vi "Purge.vi"(5 "Digital I/O Pin":u8=7, 7 "Arduino Resource":T1={"VISA resource"="GlueCTRL", "Board Type"=enum."Uno", "Connection Type"=enum."USB / Serial", "Bytes Per Packet (15)"=15}, 8 "Pin Down?":bool=TRUE, 9 "Axis Speeds":T3={"X [mm/s]"=25.0, "Y [mm/s]"=25.0, "Z [mm/s]"=10.0}, 10 "Start Position [mm]":dbl[](array[numeric]), 11 ".NET Refnum In":refnum<k24>) -> ()   [LabVIEW 2016]
uses:
  C:/Users/Aerotech/Documents/BNLStaveAssembly-blueprint/Bin/Aerotech.A3200.dll
  BNLStaveAssembly-blueprint/Bin/Aerotech.A3200.dll
  <vilib>/LabVIEW Interface for Arduino/Type Defs/Arduino Resource.ctl
  <vilib>/LabVIEW Interface for Arduino/Type Defs/Board Type.ctl
  <vilib>/LabVIEW Interface for Arduino/LabVIEW Interface for Arduino.lvlib
panel:
  in  "Absolute Purge Height [mm]":dbl=-30.0 format="%#_13g"
  in  "Relative Change in X, Y to Purge [mm]":dbl[](array[numeric])=[0.0, -150.0, 0.0]
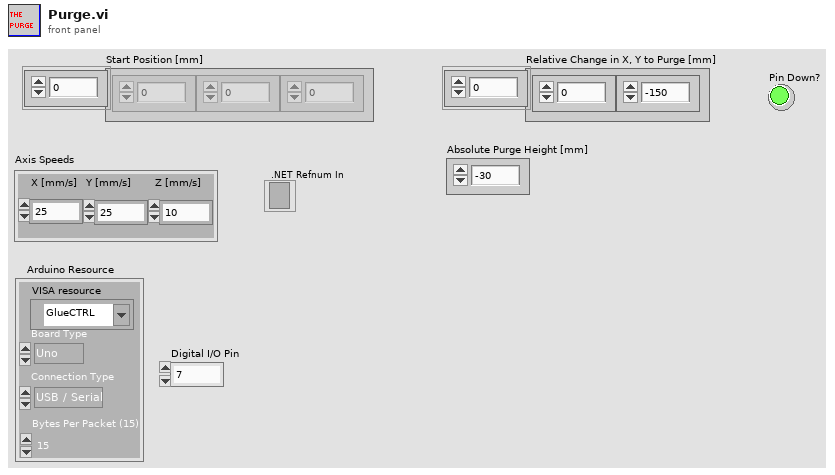
[diagram p1: front panel]
types:
  T1 = typedef "LabVIEW Interface for Arduino.lvlib/Arduino Resource.ctl" = cluster{"VISA resource":refnum<visa-resource-name>, "Board Type":T2, "Connection Type":enum8{"USB / Serial"}, "Bytes Per Packet (15)":u8}
  T2 = typedef "LabVIEW Interface for Arduino.lvlib/Board Type.ctl" = enum16{"Uno", "Dimuelanove w/Atmega 328", "Mega 2560"}
  T3 = cluster{"X [mm/s]":dbl, "Y [mm/s]":dbl, "Z [mm/s]":dbl}
  T4 = cluster{"Start Position [mm][0]":dbl, "Start Position [mm][1]":dbl, "Start Position [mm][2]":dbl}
  T5 = cluster{"Final X":dbl, "Final Y":dbl, "Final Z":dbl}
  T6 = cluster{"Final Position[0]":dbl, "Final Position[1]":dbl, "Final Position[2]":dbl}
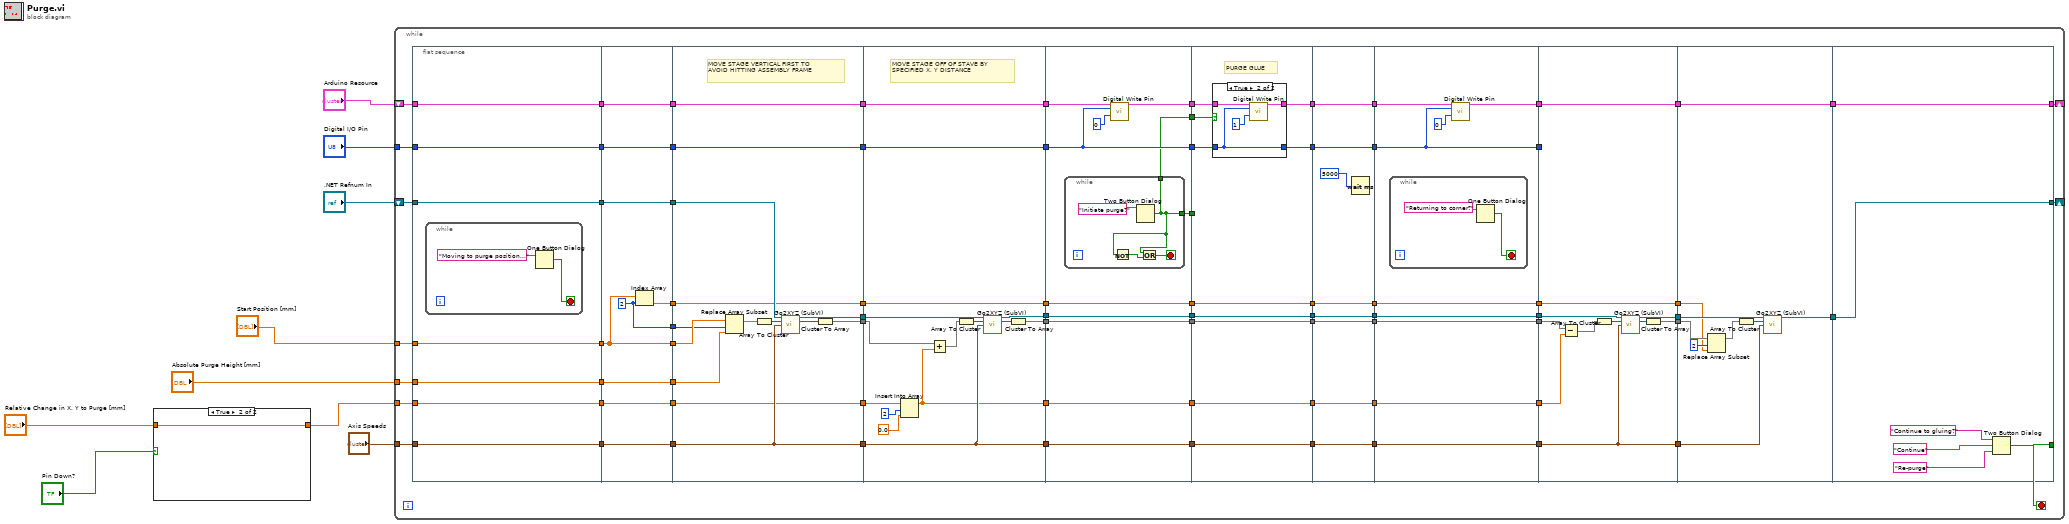
[diagram p0: block diagram]
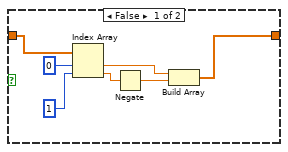
[diagram p2: hidden frame]
diagram:
  n1 = case shown="True" "Pin Down?" {
    tunnel: "Relative Change in X, Y to Purge [mm]" -> [w16 w17]
    tunnel: [w10 w17] -> w1
    frame False {
      n2 = Index Array(array=w16, index #1=0 ("index"), index #2=1 ("index")) -> (element #1=w12:dbl, element #2=w13:dbl)
      n3 = Negate(x=w13) -> (-x=w11:dbl)
      n4 = Build Array(w12, w11) -> (w10:dbl[])
    }
    frame True {
    }
  }
  n5 = while {
    tunnel: "Start Position [mm]" -> [w93]
    tunnel: w1 -> [w92]
    tunnel: "Axis Speeds" -> [w91]
    shift-right: [w87] -> _
    shift-left: ".NET Refnum In" -> [w90]
    tunnel: "Digital I/O Pin" -> [w85]
    shift-right: [w80] -> _
    shift-left: "Arduino Resource" -> [w86]
    tunnel: "Absolute Purge Height [mm]" -> [w57]
    stop <- w94 stop-if-true
    n6 = flat-sequence {
      tunnel: [w101] -> w33
      tunnel: w93 -> [w101]
      tunnel: w92 -> [w100]
      tunnel: [w100] -> w31
      tunnel: [w99] -> w29
      tunnel: w91 -> [w99]
      tunnel: [w98] -> w27
      tunnel: w90 -> [w98]
      tunnel: [w97] -> w25
      tunnel: w86 -> [w97]
      tunnel: w85 -> [w96]
      tunnel: [w96] -> w23
      tunnel: w57 -> [w95]
      tunnel: [w95] -> w21
      tunnel: w33 -> [w106]
      tunnel: [w106] -> w32
      tunnel: w31 -> [w112]
      tunnel: [w112] -> w30
      tunnel: w29 -> [w111]
      tunnel: [w111] -> w28
      tunnel: w27 -> [w110]
      tunnel: [w110] -> w26
      tunnel: w25 -> [w109]
      tunnel: [w109] -> w24
      tunnel: w23 -> [w108]
      tunnel: [w108] -> w22
      tunnel: w21 -> [w107]
      tunnel: [w107] -> w20
      tunnel: [w105] -> w19
      tunnel: [w104] -> w18
      tunnel: w32 -> [w115]
      tunnel: w30 -> [w119]
      tunnel: w28 -> [w124]
      tunnel: w26 -> [w126]
      tunnel: [w125] -> w67
      tunnel: [w124] -> w65
      tunnel: w24 -> [w123]
      tunnel: [w123] -> w63
      tunnel: w22 -> [w122]
      tunnel: [w122] -> w61
      tunnel: [w120] -> w59
      tunnel: [w119] -> w58
      tunnel: w20 -> [w117]
      tunnel: [w114] -> w40
      tunnel: w19 -> [w114]
      tunnel: w18 -> [w113]
      tunnel: w67 -> [w139]
      tunnel: [w138] -> w66
      tunnel: w65 -> [w131]
      tunnel: [w131] -> w64
      tunnel: w63 -> [w141]
      tunnel: [w141] -> w62
      tunnel: w61 -> [w140]
      tunnel: [w140] -> w60
      tunnel: w59 -> [w136]
      tunnel: w58 -> [w132]
      tunnel: [w129] -> w56
      tunnel: [w128] -> w43
      tunnel: w40 -> [w127]
      tunnel: [w127] -> w39
      tunnel: [w152] -> w84
      tunnel: w66 -> [w152]
      tunnel: [w151] -> w83
      tunnel: w64 -> [w151]
      tunnel: w62 -> [w149]
      tunnel: w60 -> [w147]
      tunnel: [w148] -> w82
      tunnel: [w147] -> w79
      tunnel: [w146] -> w77
      tunnel: [w145] -> w76
      tunnel: w56 -> [w144]
      tunnel: [w144] -> w48
      tunnel: [w143] -> w44
      tunnel: w43 -> [w143]
      tunnel: w39 -> [w142]
      tunnel: [w142] -> w34
      tunnel: w84 -> [w166]
      tunnel: [w166] -> w75
      tunnel: w83 -> [w165]
      tunnel: [w165] -> w73
      tunnel: w82 -> [w164]
      tunnel: [w163] -> w71
      tunnel: [w161] -> w69
      tunnel: w79 -> [w162]
      tunnel: w77 -> [w160]
      tunnel: w76 -> [_]
      tunnel: [w159] -> w49
      tunnel: w48 -> [w159]
      tunnel: [w158] -> w45
      tunnel: w44 -> [w158]
      tunnel: [w157] -> w35
      tunnel: w34 -> [w157]
      tunnel: w75 -> [w180]
      tunnel: [w180] -> w74
      tunnel: w73 -> [w179]
      tunnel: [w179] -> w72
      tunnel: w71 -> [w178]
      tunnel: [w178] -> w70
      tunnel: w69 -> [w177]
      tunnel: [w177] -> w68
      tunnel: [w175] -> w50
      tunnel: w49 -> [w175]
      tunnel: [w174] -> w46
      tunnel: w45 -> [w174]
      tunnel: [w173] -> w36
      tunnel: w35 -> [w173]
      tunnel: w74 -> [w189]
      tunnel: [w189] -> w89
      tunnel: w72 -> [w188]
      tunnel: [w188] -> w88
      tunnel: w70 -> [w186]
      tunnel: [w185] -> w81
      tunnel: w68 -> [w184]
      tunnel: [w184] -> w78
      tunnel: [w183] -> w51
      tunnel: w50 -> [w183]
      tunnel: [w182] -> w47
      tunnel: w46 -> [w182]
      tunnel: [w181] -> w37
      tunnel: w36 -> [w181]
      tunnel: w89 -> [w201]
      tunnel: w88 -> [w193]
      tunnel: [w200] -> w55
      tunnel: [w199] -> w53
      tunnel: w81 -> [w199]
      tunnel: w78 -> [_]
      tunnel: w51 -> [w198]
      tunnel: w47 -> [w196]
      tunnel: [w194] -> w42
      tunnel: [w193] -> w41
      tunnel: [w192] -> w38
      tunnel: w37 -> [w192]
      tunnel: w55 -> [w210]
      tunnel: [w209] -> w54
      tunnel: w53 -> [w211]
      tunnel: [w211] -> w52
      tunnel: w42 -> [w206]
      tunnel: w41 -> [w207]
      tunnel: w38 -> [w204]
      tunnel: [w216] -> w94
      tunnel: w54 -> [w215]
      tunnel: [w215] -> w87
      tunnel: [w214] -> w80
      tunnel: w52 -> [w214]
      frame #0 {
        n7 = while {
          stop <- w102 stop-if-true
          n8 = One Button Dialog(message="Moving to purge position...") -> (true=w102:bool)  [unwired: 1 in]
        }
      }
      frame #1 {
        w104 = 2 ("index")
        n9 = Index Array(array=w106, index=w104) -> (element=w105:dbl)
      }
      frame #2 {
        # "MOVE STAGE VERTICAL FIRST TO\nAVOID HITTING ASSEMBLY FRAME"
        n10 = Replace Array Subset(array=w115, new element=w117, index=w113) -> (w116:dbl[])
        n11 = Array To Cluster(array=w116) -> (cluster=w118:T4)
        n12 = call "Go2XYZ (SubVI).vi"(".NET Refnum in"=w126, "Go to Coordinates"=w118, "Axis Speeds"=w124) -> (".NET Refnum out"=w125:refnum<k24>, "Final Position"=w121:T5)  [unwired: 8 in, 3 out]
        n13 = Cluster To Array(cluster=w121) -> (array=w120:dbl[])
      }
      frame #3 {
        # "MOVE STAGE OFF OF STAVE BY\nSPECIFIED X, Y DISTANCE"
        n14 = Insert Into Array(array=w132, index=2, new element=0.0 ("new element/subarray")) -> (w128:dbl[])
        n15 = Add(x=w136, y=w128) -> (x+y=w135:dbl[])
        n16 = Array To Cluster(array=w135) -> (cluster=w137:cluster{"[0]":dbl, "[1]":dbl, "[2]":dbl})
        n17 = call "Go2XYZ (SubVI).vi"(".NET Refnum in"=w139, "Go to Coordinates"=w137, "Axis Speeds"=w131) -> (".NET Refnum out"=w138:refnum<k24>, "Final Position"=w130:T5)  [unwired: 8 in, 3 out]
        n18 = Cluster To Array(cluster=w130) -> (array=w129:dbl[])
      }
      frame #4 {
        n19 = while {
          tunnel: [w153] -> w146
          tunnel: [w153] -> w145
          stop <- w154 stop-if-true
          n20 = Two Button Dialog(message="Initiate purge?") -> (T button?=w153:bool)  [unwired: 2 in]
          n21 = Not(x=w153) -> (.not. x?=w155:bool)
          n22 = Or(x=w153, y=w155) -> (x .or. y?=w154:bool)
        }
        n23 = call <vilib>:"Digital Write Pin.vi"("Arduino Resource"=w149, "Digital I/O Pin (0)"=w147, "Value (0)"=u8 0) -> ("Arduino Resource"=w148:T1)  [unwired: 11 in, 1 out]
      }
      frame #5 {
        # "PURGE GLUE"
        n24 = case shown="True" w160 {
          tunnel: w164 -> [w167 w171]
          tunnel: [w167 w170] -> w163
          tunnel: w162 -> [w168 w169]
          tunnel: [w168 w169] -> w161
          frame False {
          }
          frame True {
            n25 = call <vilib>:"Digital Write Pin.vi"("Arduino Resource"=w171, "Digital I/O Pin (0)"=w169, "Value (0)"=u8 1) -> ("Arduino Resource"=w170:T1)  [unwired: 11 in, 1 out]
          }
        }
      }
      frame #6 {
        n26 = Wait (ms)(milliseconds to wait=u32 5000) -> ()  [unwired: 1 out]
      }
      frame #7 {
        n27 = while {
          stop <- w191 stop-if-true
          n28 = One Button Dialog(message="Returning to corner?") -> (true=w191:bool)  [unwired: 1 in]
        }
        n29 = call <vilib>:"Digital Write Pin.vi"("Arduino Resource"=w186, "Digital I/O Pin (0)"=w184, "Value (0)"=u8 0) -> ("Arduino Resource"=w185:T1)  [unwired: 11 in, 1 out]
      }
      frame #8 {
        n30 = Subtract(x=w198, y=w196) -> (x-y=w197:dbl[])
        n31 = Array To Cluster(array=w197) -> (cluster=w202:cluster{"[0]":dbl, "[1]":dbl, "[2]":dbl})
        n32 = call "Go2XYZ (SubVI).vi"(".NET Refnum in"=w201, "Go to Coordinates"=w202, "Axis Speeds"=w193) -> (".NET Refnum out"=w200:refnum<k24>, "Final Position"=w195:T5)  [unwired: 8 in, 3 out]
        n33 = Cluster To Array(cluster=w195) -> (array=w194:dbl[])
      }
      frame #9 {
        n34 = Replace Array Subset(array=w206, new element=w204, index=2) -> (w203:dbl[])
        n35 = Array To Cluster(array=w203) -> (cluster=w208:T6)
        n36 = call "Go2XYZ (SubVI).vi"(".NET Refnum in"=w210, "Go to Coordinates"=w208, "Axis Speeds"=w207) -> (".NET Refnum out"=w209:refnum<k24>)  [unwired: 8 in, 4 out]
      }
      frame #10 {
        n37 = Two Button Dialog(message="Continue to gluing?", 1:"Re-purge" ("F button name (\"Cancel\")"), 2:"Continue" ("T button name (\"OK\")")) -> (T button?=w216:bool)
      }
    }
  }
